vi "Add Service.vi"(8 "error in (no error)":errorcluster, 10 "Service.lvclass":refnum<class "Service.lvclass">, 11 "Server in":refnum<class "Server.lvclass">) -> (0 "error out":errorcluster, 3 "Server out":refnum<class "Server.lvclass">)   [LabVIEW 2024, in "Ramses Framework.lvlib" / "Server.lvclass"]
doc: "Register a service with the server instance."
uses:
  Server.lvclass
  Service/Service.lvclass
  Server.lvclass/Server.ctl
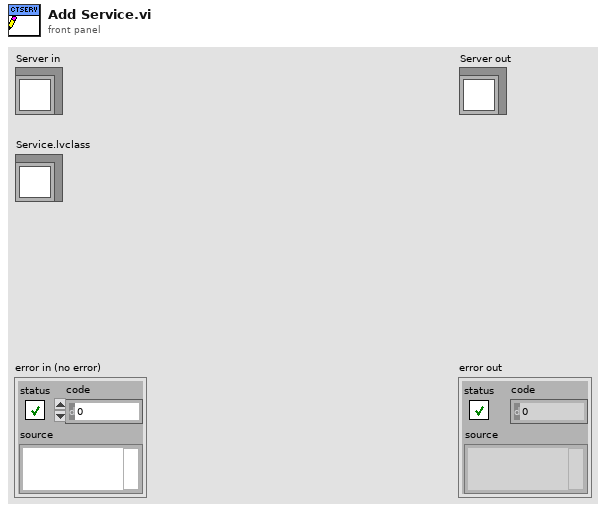
[diagram p1: front panel]
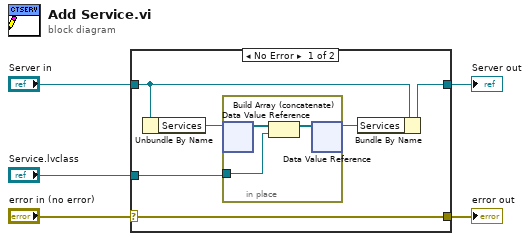
[diagram p0: block diagram]
diagram:
  n1 = case shown="No Error" "error in (no error)" {
    selector: "error in (no error)" -> [w11 w15]
    tunnel: [w11 w15] -> w4
    tunnel: [w10 w16] -> w2
    tunnel: "Server in" -> [w9 w16]
    tunnel: "Service.lvclass" -> [w8 _]
    frame No Error {
      n2 = Unbundle By Name(w9) -> ("Services"=w7:refnum<data-value>)
      n3 = in-place {
        in-place-border: w8 -> [w14]
        n4 = in-place-dvr #1(w7) -> (w13:refnum<class "Service.lvclass">[])  [unwired: 1 out]
        n5 = Build Array (concatenate)(w13, w14) -> (w12:refnum<class "Service.lvclass">[])
        n6 = in-place-dvr #1(w12) -> (w6:refnum<data-value>)  [unwired: 1 out]
      }
      n7 = Bundle By Name(cluster=w9, "Services"=w6) -> (w10:refnum<class "Server.lvclass">)
    }
    frame Error {
    }
  }
  "error out" <- w4
  "Server out" <- w2
